vi "Add to OPC UA Server.vi"(8 "Error In":errorcluster, 10 "OPC UA server refnum in":refnum<k21>, 11 "Sync Tag In":refnum<class "Synchronised Tag.lvclass">) -> (0 "error out":errorcluster, 1 "URL":string, 2 "OPC UA server refnum out":refnum<k21>, 3 "Sync Tag Out":refnum<class "Synchronised Tag.lvclass">)   [LabVIEW 2016, in "Synchronised Tag.lvclass"]
uses:
  Synchronised Tag.lvclass
  Controls/OPC type.ctl
  <vilib>/OPCUA/NI OPC UA Server.lvlib
  <vilib>/OPCUA/NI OPC UA Utility.lvlib
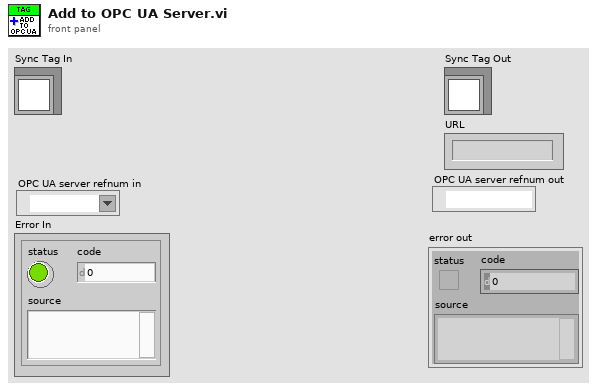
[diagram p1: front panel]
types:
  T1 = typedef "Node Type.ctl" = enum16{"Property", "Item", "Folder"}
  T2 = typedef "SV type.ctl" = enum16{"Boolean", "SByte", "Byte", "Int16", "UInt16", "Int32", "UInt32", "Int64", "UInt64", "Float", "Double", "String", "DateTime", "ByteString", "Array of Boolean", "Array of SByte", "Array of Byte", "Array of Int16", "Array of UInt16", "Array of Int32", "Array of UInt32", "Array of Int64", "Array of UInt64", "Array of Float", "Array of Double", "Array of String", "Array of DateTime", "Array of ByteString", "Unsupported"}
  T3 = typedef "OPC type.ctl" = u16
  T4 = typedef "Synchronised Tag.lvclass/Access Mode.ctl" = enum16{"Unused", "Read Only", "Write Only", "Read/Write"}
  T5 = cluster{"name":string, "data type":u16, "access level":u16, "description":string}
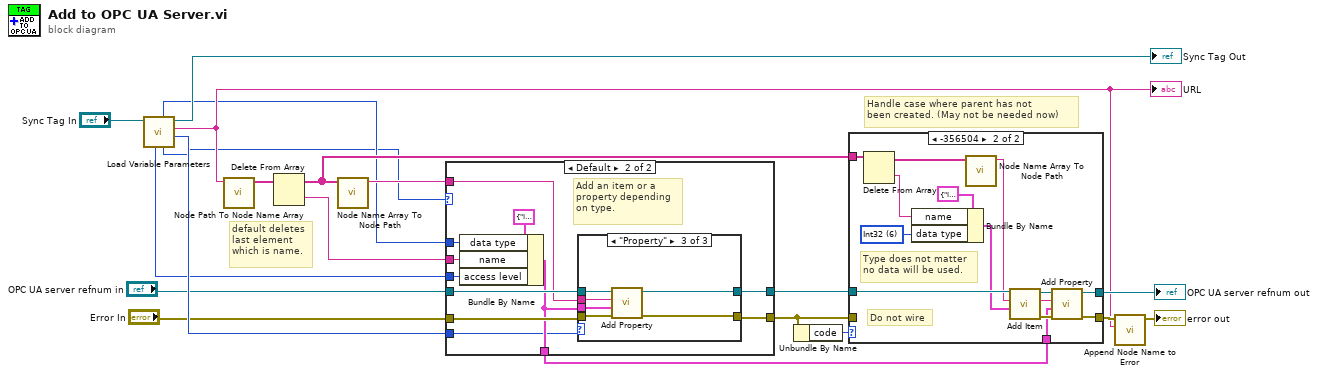
[diagram p0: block diagram]
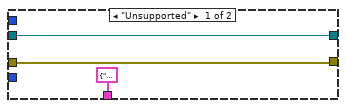
[diagram p2: hidden frame]
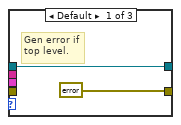
[diagram p3: hidden frame]
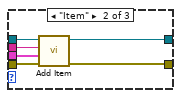
[diagram p4: hidden frame]
diagram:
  # "Handle case where parent has not\nbeen created. (May not be needed now)"
  # "default deletes\nlast element\nwhich is name."
  n1 = call "Load Variable Parameters.vi"("Sync Tag In"="Sync Tag In") -> ("Node Type"=w11:T1, "URL"=w5:string, "Sync Tag Out"=→"Sync Tag Out":refnum<class "Synchronised Tag.lvclass">, "SV Data Type"=w3:T2, "OPC UA type"=w4:T3, "Access Mode"=w2:T4)  [unwired: 4 in, 1 out]
  "URL" <- w5
  n2 = call <vilib>:"Node Path To Node Name Array.vi"("node path"=w5) -> ("node names"=w20:string[])  [unwired: 9 in, 1 out]
  n3 = Delete From Array(array=w20) -> (deleted portion=w18:string, array with subset deleted=w13:string[])  [unwired: 2 in]
  n4 = call <vilib>:"Node Name Array To Node Path.vi"("node names"=w13) -> ("node path"=w19:string)  [unwired: 9 in, 1 out]
  n5 = case shown="Default" w3 {
    tunnel: "OPC UA server refnum in" -> [w23 w34]
    tunnel: "Error In" -> [w22 w33]
    tunnel: w19 -> [_ w32]
    tunnel: w4 -> [_ w30]
    tunnel: w18 -> [_ w29]
    tunnel: [w22 w28] -> w15
    tunnel: [w23 w27] -> w14
    tunnel: [T5 {"name"="", "data type"=0, "access level"=0, "description"=""} ("item") w26] -> w12
    tunnel: w11 -> [_ w25]
    tunnel: w2 -> [_ w24]
    frame "Unsupported" {
    }
    frame Default {
      # "Add an item or a\nproperty depending\non type."
      n6 = Bundle By Name(cluster=T5 {"name"="Int32Node", "data type"=6, "access level"=3, "description"=""} ("item"), "data type"=w30, "name"=w29, "access level"=w24) -> (w26:T5)
      n7 = case shown="\"Property\"" w25 {
        tunnel: w34 -> [w36 w42 w48]
        tunnel: w33 -> [_ w41 w47]
        tunnel: w32 -> [_ w40 w46]
        tunnel: w26 -> [_ w39 w45]
        tunnel: [w36 w38 w44] -> w27
        tunnel: [errorcluster {"status"=TRUE, "code"=-356506, "source"=""} ("error out") w37 w43] -> w28
        frame Default {
          # "Gen error if\ntop level."
        }
        frame "Item" {
          n8 = call <vilib>:"Add Item.vi"("error in (no error)"=w41, "item"=w39, "parent folder path"=w40, "OPC UA server refnum in"=w42) -> ("error out"=w37:errorcluster, "OPC UA server refnum out"=w38:refnum<k21>)  [unwired: 4 in, 1 out]
        }
        frame "Property" {
          n9 = call <vilib>:"Add Property.vi"("error in (no error)"=w47, "property"=w45, "item path"=w46, "OPC UA server refnum in"=w48) -> ("error out"=w43:errorcluster, "OPC UA server refnum out"=w44:refnum<k21>)  [unwired: 4 in, 1 out]
        }
      }
    }
  }
  n10 = Unbundle By Name(w15) -> ("code"=w17:i32)
  n11 = case shown="-356504" w17 {
    tunnel: [w50 w56] -> w16
    tunnel: w15 -> [w50 _]
    tunnel: w14 -> [w49 w64]
    tunnel: w13 -> [_ w63]
    tunnel: w12 -> [_ w57]
    tunnel: [w49 w55] -> w7
    frame 0, Default {
    }
    frame -356504 {
      w52 = T3 6 items=["Boolean"=1, "SByte"=2, "Byte"=3, "Int16"=4, "UInt16"=5, "Int32"=6, "UInt32"=7, "Int64"=8, "UInt64"=9, "Float"=10, "Double"=11, "String"=12, "DateTime"=13, "ByteString"=15, "Array of Boolean"=101, "Array of SByte"=102, "Array of Byte"=103, "Array of Int16"=104, "Array of UInt16"=105, "Array of Int32"=106, "Array of UInt32"=107, "Array of Int64"=108, "Array of UInt64"=109, "Array of Float"=110, "Array of Double"=111, "Array of String"=112, "Array of DateTime"=113, "Array of ByteString"=115] ("OPC type")
      # "Do not wire"
      # "Type does not matter\nno data will be used."
      n12 = Delete From Array(array=w63) -> (deleted portion=w53:string, array with subset deleted=w62:string[])  [unwired: 2 in]
      n13 = Bundle By Name(cluster=T5 {"name"="Int32Node", "data type"=6, "access level"=3, "description"=""} ("item"), "name"=w53, "data type"=w52) -> (w51:T5)
      n14 = call <vilib>:"Node Name Array To Node Path.vi"("node names"=w62) -> ("node path"=w61:string)  [unwired: 9 in, 1 out]
      n15 = call <vilib>:"Add Item.vi"("item"=w51, "parent folder path"=w61, "OPC UA server refnum in"=w64) -> ("error out"=w60:errorcluster, "item path"=w59:string, "OPC UA server refnum out"=w58:refnum<k21>)  [unwired: 5 in]
      n16 = call <vilib>:"Add Property.vi"("error in (no error)"=w60, "property"=w57, "item path"=w59, "OPC UA server refnum in"=w58) -> ("error out"=w56:errorcluster, "OPC UA server refnum out"=w55:refnum<k21>)  [unwired: 4 in, 1 out]
    }
  }
  "OPC UA server refnum out" <- w7
  n17 = call "Append Node Name to Error.vi"("Node Name"=w5, "error in (no error)"=w16) -> ("error out"=→"error out":errorcluster)  [unwired: 9 in]
